vi "HEWH Cut Power.vi"(9 "Cut Power At Time (Sec)":T1 format="%<%H:%M:%S>t", 10 "Current Draw Time (Sec)":T1 format="%<%H:%M:%S>t", 11 "User Controls in":T2={"Main Power Control"=FALSE, "Flow Totalizer Control"=FALSE, "Intellifaucet Temperature"=0.0, "Percent Flow"=0.0, "Safe Mode"=FALSE, "GEA2?"=FALSE, "Use Agilent?"=FALSE, "Valve Set A"=enum."Heating", "Valve Set B"=enum."Heating", "Valve Set C"=enum."Heating", "Valve Set D"=enum."Heating", "Valves"={"In VLV A"=enum."OPEN", "Drain VLV A"=enum."OPEN", "Out VLV A"=enum."CLOSE", "In VLV B"=enum."OPEN", "Drain VLV B"=enum."OPEN", "Out VLV B"=enum."CLOSE", "In VLV C"=enum."OPEN", "Drain VLV C"=enum."OPEN", "Out VLV C"=enum."CLOSE", "In VLV D"=enum."OPEN", "Drain VLV D"=enum."OPEN", "Out VLV D"=enum."CLOSE"}} {"Percent Flow" scale=40.0..120.0; "Intellifaucet Temperature" scale=40.0..120.0}) -> (2 "States Output":string, 3 "User Controls out":T2={"Main Power Control"=FALSE, "Flow Totalizer Control"=FALSE, "Intellifaucet Temperature"=0.0, "Percent Flow"=0.0, "Safe Mode"=FALSE, "GEA2?"=FALSE, "Use Agilent?"=FALSE, "Valve Set A"=enum."Heating", "Valve Set B"=enum."Heating", "Valve Set C"=enum."Heating", "Valve Set D"=enum."Heating", "Valves"={"In VLV A"=enum."OPEN", "Drain VLV A"=enum."OPEN", "Out VLV A"=enum."CLOSE", "In VLV B"=enum."OPEN", "Drain VLV B"=enum."OPEN", "Out VLV B"=enum."CLOSE", "In VLV C"=enum."OPEN", "Drain VLV C"=enum."OPEN", "Out VLV C"=enum."CLOSE", "In VLV D"=enum."OPEN", "Drain VLV D"=enum."OPEN", "Out VLV D"=enum."CLOSE"}} {"Percent Flow" scale=40.0..120.0; "Intellifaucet Temperature" scale=40.0..120.0})   [LabVIEW 2016]
uses:
  Type Definitions/HEWH User Controls.ctl
  Custom Instrument Control/MW100/Type Definitions/HEWH Solenoid Valve Status.ctl
  Utility/Custom Pallet Controls/Custom Pallet Timer.ctl
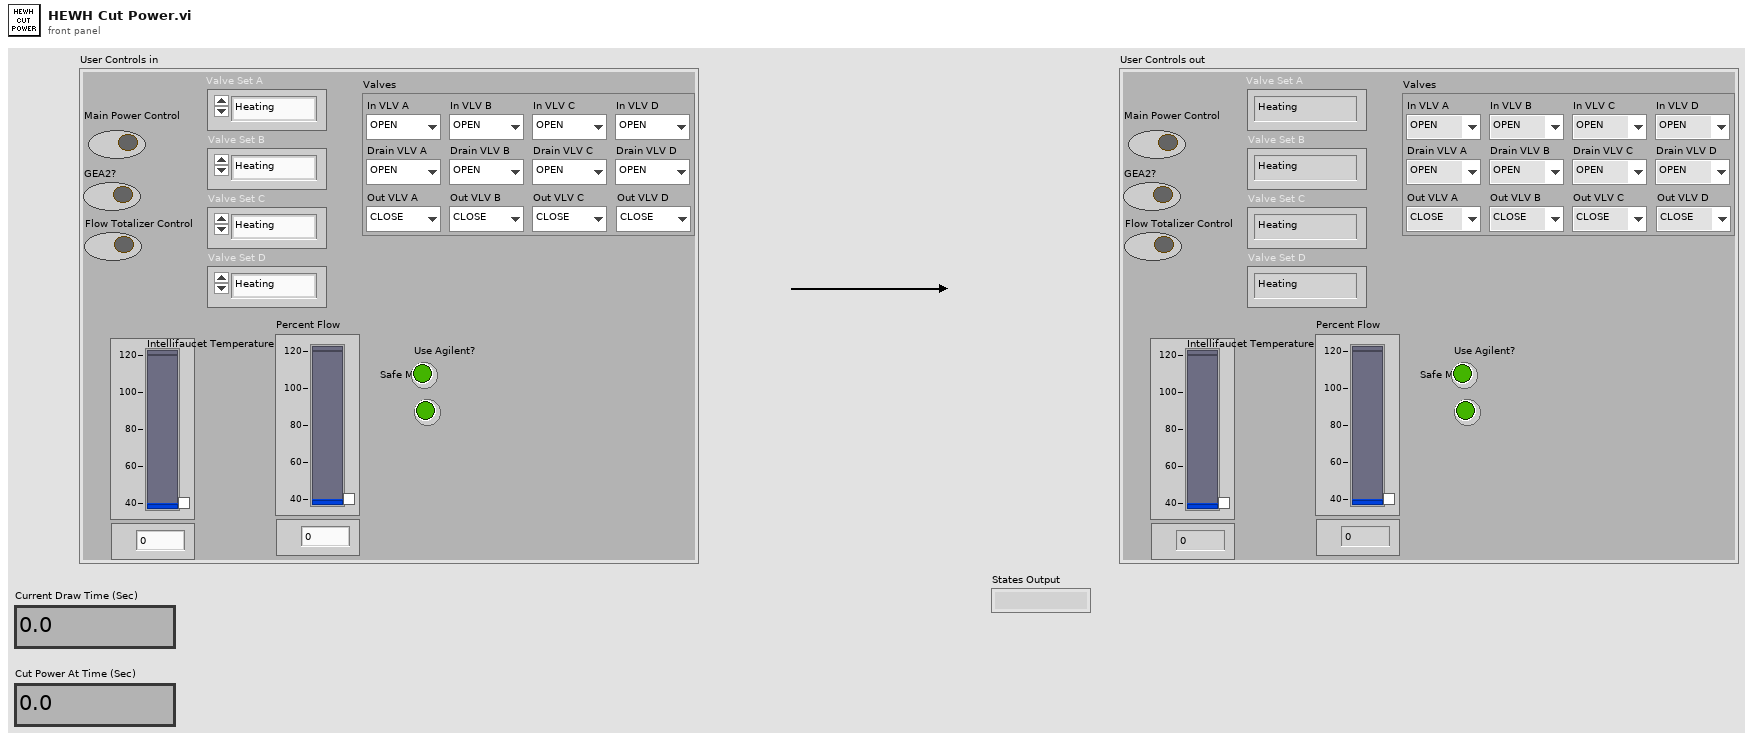
[diagram p1: front panel]
types:
  T1 = typedef "Custom Pallet Timer.ctl" = dbl
  T2 = typedef "HEWH User Controls.ctl" = cluster{"Main Power Control":bool, "Flow Totalizer Control":bool, "Intellifaucet Temperature":dbl, "Percent Flow":dbl, "Safe Mode":bool, "GEA2?":bool, "Use Agilent?":bool, "Valve Set A":enum16{"Heating", "Purge", "Resting", "Draw"}, "Valve Set B":enum16{"Heating", "Purge", "Resting", "Draw"}, "Valve Set C":enum16{"Heating", "Purge", "Resting", "Draw"}, "Valve Set D":enum16{"Heating", "Purge", "Resting", "Draw"}, "Valves":cluster{"In VLV A":T3, "Drain VLV A":T3, "Out VLV A":T3, "In VLV B":T3, "Drain VLV B":T3, "Out VLV B":T3, "In VLV C":T3, "Drain VLV C":T3, "Out VLV C":T3, "In VLV D":T3, "Drain VLV D":T3, "Out VLV D":T3}}
  T3 = typedef "HEWH Solenoid Valve Status.ctl" = enum8{"CLOSE", "OPEN"}
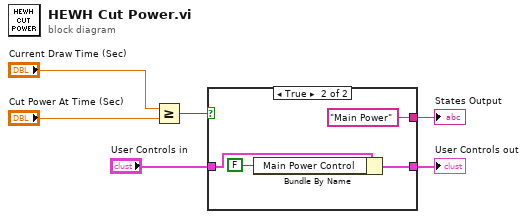
[diagram p0: block diagram]
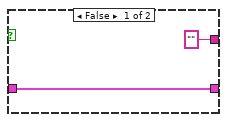
[diagram p2: hidden frame]
diagram:
  n1 = Greater Or Equal?(x="Current Draw Time (Sec)", y="Cut Power At Time (Sec)") -> (x >= y?=w3:bool)
  n2 = case shown="True" w3 {
    tunnel: ["" ("State(s) in Front (\"\")") "Main Power" ("State(s) in Front (\"\")")] -> w4
    tunnel: "User Controls in" -> [w7 w11]
    tunnel: [w7 w10] -> w6
    frame False {
    }
    frame True {
      n3 = Bundle By Name(cluster=w11, "Main Power Control"=FALSE ("User Controls.Main Power Control")) -> (w10:T2)
    }
  }
  "User Controls out" <- w6
  "States Output" <- w4
